vi "Demo_1.vi"() -> ()   [LabVIEW 2017]
uses:
  Components/ViPER.lvlibp/ViPER.lvclass
panel:
  in  "Path":path
  out "error out":errorcluster
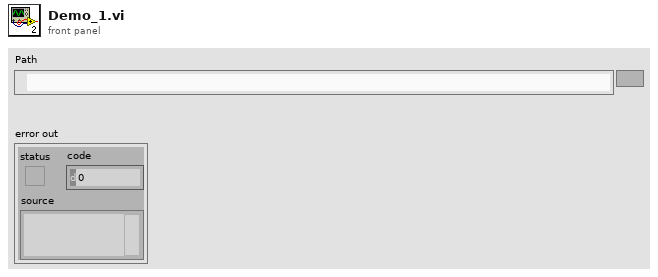
[diagram p1: front panel]
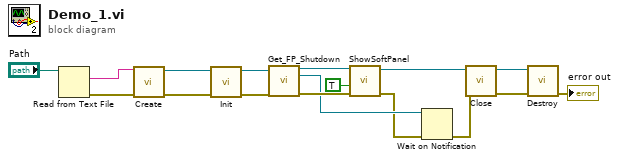
[diagram p0: block diagram]
diagram:
  n1 = Read from Text File(file (use dialog)="Path") -> (text=w1:string, error out=w2:errorcluster)  [unwired: 3 in, 2 out]
  n2 = call "Create.vi"("error in (no error)"=w2, "Config XML"=w1) -> ("error out"=w17:errorcluster, "reference out"=w16:refnum<class "ViPER.lvclass">)  [unwired: 8 in]
  n3 = call-dynamic "Init.vi"("error in (no error)"=w17, "reference in"=w16) -> ("error out"=w15:errorcluster, "reference out"=w14:refnum<class "ViPER.lvclass">)  [unwired: 8 in]
  n4 = call "Get_FP_Shutdown.vi"("ViKing_Base in"=w14, "error in (no error)"=w15) -> ("ViKing_Base out"=w12:refnum<class "ViPER.lvclass">, "SoftFP_Shutdown"=w8:refnum<notifier>, "error out"=w13:errorcluster)  [unwired: 9 in, 2 out]
  n5 = call-dynamic "ShowSoftPanel.vi"("error in (no error)"=w13, "Floating"=TRUE, "Driver in"=w12) -> ("error out"=w4:errorcluster, "Driver out"=w6:refnum<class "ViPER.lvclass">)  [unwired: 6 in, 1 out]
  n6 = Wait on Notification(notifier=w8, error in (no error)=w4) -> (error out=w7:errorcluster)  [unwired: 2 in, 3 out]
  n7 = call-dynamic "Close.vi"("error in (no error)"=w7, "reference in"=w6) -> ("error out"=w11:errorcluster, "reference out"=w10:refnum<class "ViPER.lvclass">)  [unwired: 8 in]
  n8 = call "Destroy.vi"("error in (no error)"=w11, "reference in"=w10) -> ("error out"=→"error out":errorcluster)  [unwired: 9 in]
